vi "UpdateInventory.vi"(8 "error in (no error)":errorcluster, 11 "Coca Actors in":refnum<class "Coca Actors.lvclass">) -> (0 "error out":errorcluster, 3 "Coca Actors out":refnum<class "Coca Actors.lvclass">)   [LabVIEW 2020, in "Coca Actors.lvlib" / "Coca Actors.lvclass"]
uses:
  Coca Actors.lvclass
  Coca Actors.lvclass/Coca Actors.ctl
  <vilib>/Utility/config.llb/Read Key (Double).vi
  <vilib>/Utility/config.llb/Read Key (String).vi
  <vilib>/Utility/config.llb/NI_LVConfig.lvlib
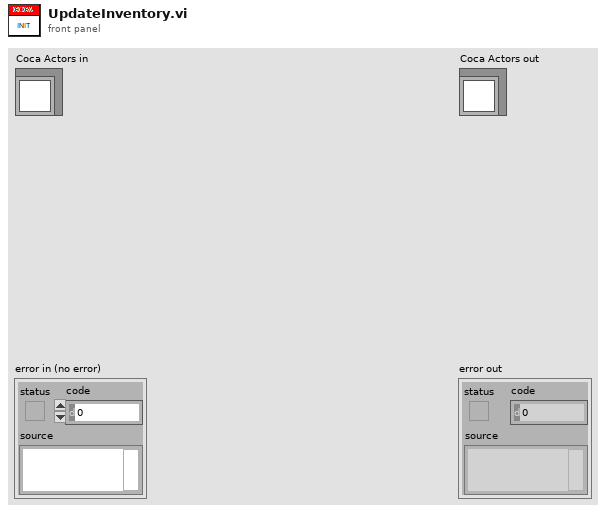
[diagram p1: front panel]
types:
  T1 = typedef "NI_LVConfig.lvlib/Config Data RefNum.ctl" = refnum<k1>
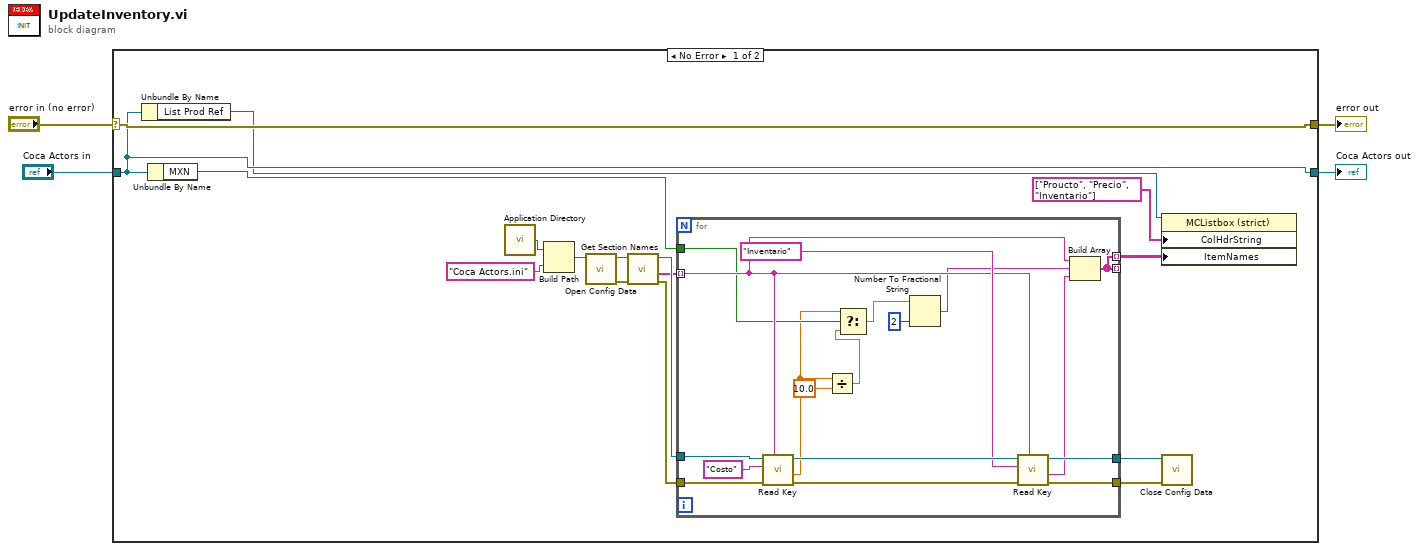
[diagram p0: block diagram]
diagram:
  n1 = case shown="No Error" "error in (no error)" {
    selector: "error in (no error)" -> [w20 w40]
    tunnel: [w20 w40] -> w3
    tunnel: [w13 w39] -> w1
    tunnel: "Coca Actors in" -> [w13 w39]
    frame No Error {
      n2 = Unbundle By Name(w13) -> ("List Prod Ref"=w7:refnum<vi>)
      n3 = Unbundle By Name(w13) -> ("MXN"=w12:bool)
      n4 = call <vilib>:"Application Directory.vi"() -> ("Application Directory"=w18:path)
      n5 = Build Path(base path=w18, name or relative path="Coca Actors.ini") -> (appended path=w17:path)
      n6 = call <vilib>:"Open Config Data.vi"("configuration file path"=w17) -> ("error out"=w16:errorcluster, "refnum"=w10:T1)  [unwired: 8 in, 1 out]
      n7 = call <vilib>:"Get Section Names.vi"("error in (no error)"=w16, "refnum"=w10) -> ("error out"=w11:errorcluster, "section names"=w8:string[], "refnum out"=w9:T1)  [unwired: 7 in]
      n8 = for {
        tunnel: w9 -> [w38]
        tunnel: w11 -> [w37]
        tunnel: [w33] -> w15
        tunnel: [w34] -> w14
        tunnel: w12 -> [w25]
        tunnel: w8 -> [w30] mode=indexing
        tunnel: [w28] -> _ mode=indexing
        tunnel: [w28] -> w6 mode=indexing
        n9 = call-poly <vilib>:"Read Key.vi"("section"=w30, "error in (no error)"=w37, "key"="Costo", "refnum"=w38) -> ("error out"=w35:errorcluster, "value"=w23:dbl, "refnum out"=w36:T1)  [unwired: 4 in, 1 out]
        n10 = Divide(x=w23, y=10.0) -> (x/y=w21:dbl)
        n11 = Select(t=w23, s=w25, f=w21) -> (s? t:f=w24:dbl)
        n12 = Number To Fractional String(number=w24, precision (6)=i16 2) -> (F-format string=w26:string)  [unwired: 2 in]
        n13 = call-poly <vilib>:"Read Key.vi"("section"=w30, "error in (no error)"=w35, "key"="Inventario", "refnum"=w36) -> ("error out"=w33:errorcluster, "value"=w29:string, "refnum out"=w34:T1)  [unwired: 4 in, 1 out]
        n14 = Build Array(w30, w26, w29) -> (w28:string[])
      }
      n15 = property class="MCListbox (strict)"(reference=w7, "ColHdrString"=string[] ["Proucto", "Precio", "Inventario"] ("Column Header Strings[]"), "ItemNames"=w6) -> ()  [unwired: 1 in, 2 out]
      n16 = call <vilib>:"Close Config Data.vi"("error in (no error)"=w15, "refnum"=w14) -> ()  [unwired: 8 in, 2 out]
    }
    frame Error {
    }
  }
  "error out" <- w3
  "Coca Actors out" <- w1
